vi "SetROI.vi"(8 "error in (no error)":errorcluster, 10 "NewROI":T1, 11 "CameraSession in":refnum<class "CS250-CameraHardwareClass.lvclass">) -> (0 "error out":errorcluster, 3 "CameraSession out":refnum<class "CS250-CameraHardwareClass.lvclass">)   [LabVIEW 2013, in "CS250-CameraHardwareClass.lvclass"]
uses:
  CS250-CameraHardwareClass.lvclass
  CS250-CameraHardwareClass.lvclass/CS250-CameraHardwareClass.ctl
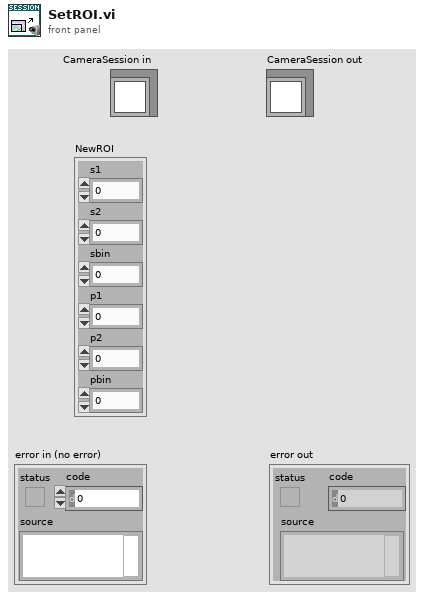
[diagram p1: front panel]
types:
  T1 = cluster{"s1":u16, "s2":u16, "sbin":u16, "p1":u16, "p2":u16, "pbin":u16}
  T2 = typedef "CamCluster.ctl" = cluster{"hcam out":i16, "TempImage":T3, "Pointer":u32, "exp_bytes out":u32, "rgn_array":cluster{"s1":u16, "s2":u16, "sbin":u16, "p1":u16, "p2":u16, "pbin":u16}, "CameraName":string}
  T3 = typedef "IMAQ Image.ctl" = refnum<image>
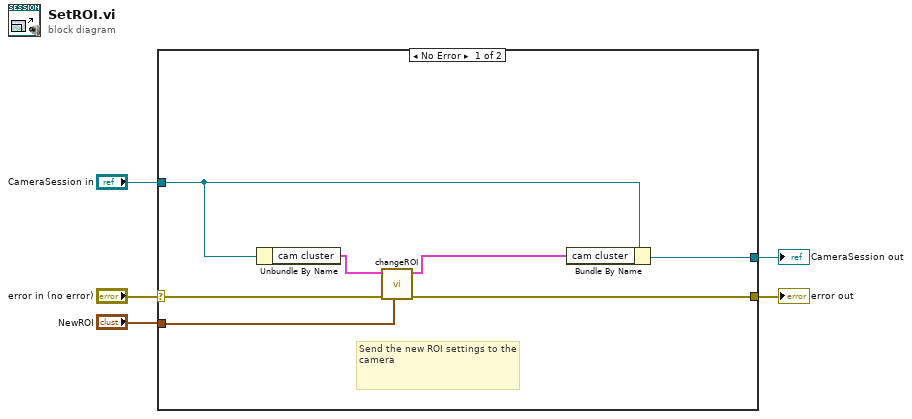
[diagram p0: block diagram]
diagram:
  n1 = case shown="No Error" "error in (no error)" {
    selector: "error in (no error)" -> [w10 w14]
    tunnel: [w9 w14] -> w4
    tunnel: [w11 w13] -> w2
    tunnel: "CameraSession in" -> [w7 w13]
    tunnel: "NewROI" -> [w6 _]
    frame No Error {
      # "Send the new ROI settings to the camera"
      n2 = Unbundle By Name(w7) -> ("cam cluster"=w12:T2)
      n3 = call "changeROI.vi"("new_rgn_array"=w6, "error in (no error)"=w10, "cam cluster out in"=w12) -> ("error out"=w9:errorcluster, "cam cluster out out"=w8:T2)  [unwired: 6 in, 1 out]
      n4 = Bundle By Name(cluster=w7, "cam cluster"=w8) -> (w11:refnum<class "CS250-CameraHardwareClass.lvclass">)
    }
    frame Error {
    }
  }
  "error out" <- w4
  "CameraSession out" <- w2
